vi "MultipleDbsPanelModel-GFV.vi"(8 "error in (no error)":errorcluster, 10 "Data in":variant, 11 "Enum":T1) -> (0 "error out":errorcluster, 3 "Data out":variant)   [LabVIEW 2013]
doc: "Use this template to build a VI to use as a subVI."
uses:
  TypeDef/MultipleFileDataModel.ctl
  TypeDef/MultipleFilesModelOutput.ctl
  TypeDef/MultipleFilesModelInput.ctl
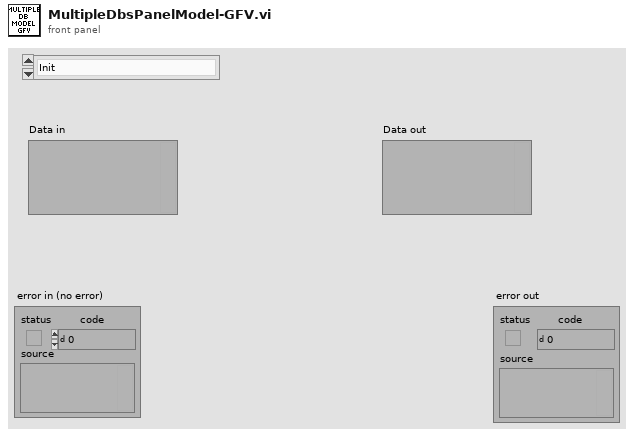
[diagram p1: front panel]
types:
  T1 = typedef "MultipleFileDataModel.ctl" = enum16{"Init", "Get Input Data", "Get Output Data", "Save Output Data", "Save Input Data"}
  T2 = typedef "MultipleFilesModelOutput.ctl" = cluster{"Ramp Pattern":dbl[], dbl[]}
  T3 = typedef "MultipleFilesModelInput.ctl" = cluster{"Min Diameter (µm)":dbl, "Max Diameter (µm)":dbl, "FilterDropletsFrozeBelow":dbl, "Temperature offset for Calibration":dbl, "BinSizeDeg":dbl}
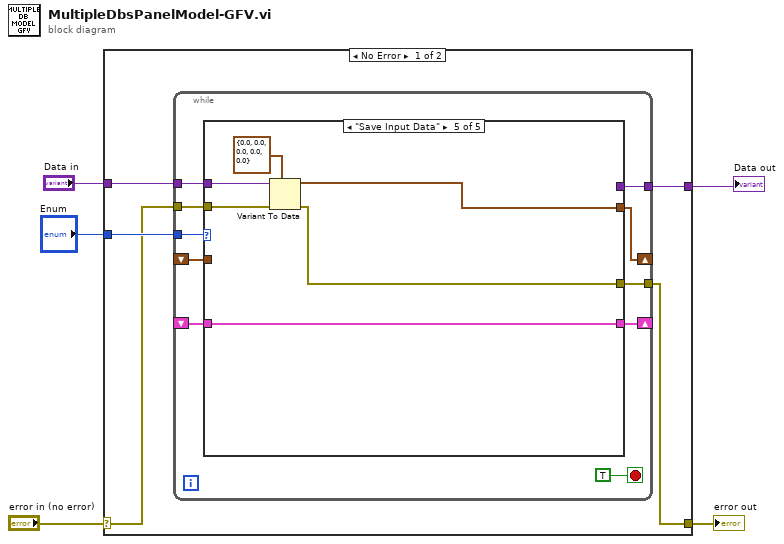
[diagram p0: block diagram]
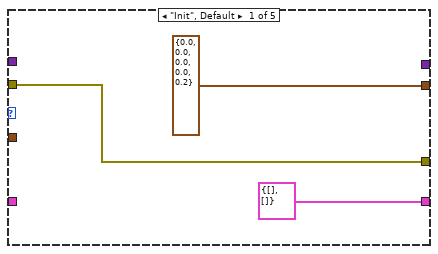
[diagram p2: hidden frame]
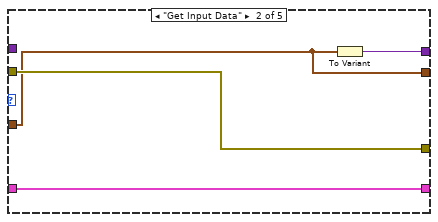
[diagram p3: hidden frame]
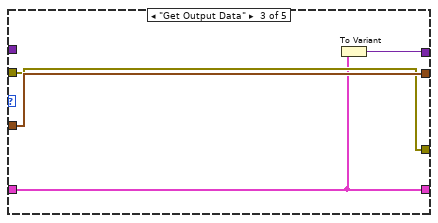
[diagram p4: hidden frame]
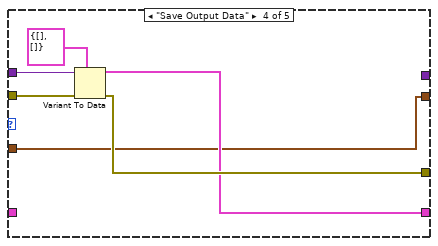
[diagram p5: hidden frame]
diagram:
  n1 = case shown="No Error" "error in (no error)" {
    selector: "error in (no error)" -> [w8 w44]
    tunnel: [w7 w44] -> w4
    tunnel: "Enum" -> [w10 _]
    tunnel: "Data in" -> [w9 _]
    tunnel: [w6 _] -> w1
    frame No Error {
      n2 = while {
        tunnel: w10 -> [w19]
        shift-right: [w18] -> _
        shift-left: _ -> [w14]
        tunnel: w9 -> [w17]
        tunnel: w8 -> [w16]
        tunnel: [w15] -> w7
        tunnel: [w13] -> w6
        shift-right: [w12] -> _
        shift-left: _ -> [w11]
        stop <- TRUE stop-if-true
        n3 = case shown="\"Save Input Data\"" w19 {
          tunnel: [T3 {"Min Diameter (µm)"=0.0, "Max Diameter (µm)"=0.0, "FilterDropletsFrozeBelow"=0.0, "Temperature offset for Calibration"=0.0, "BinSizeDeg"=0.2} w25 w31 w32 w39] -> w18
          tunnel: w17 -> [_ _ _ w37 w43]
          tunnel: w16 -> [w22 w26 w30 w36 w42]
          tunnel: [w22 w26 w30 w35 w41] -> w15
          tunnel: w14 -> [_ w25 w31 w32 _]
          tunnel: [_ w27 w29 _ _] -> w13
          tunnel: [T2 {"Ramp Pattern"=[], []} w24 w28 w33 w38] -> w12
          tunnel: w11 -> [_ w24 w28 _ w38]
          frame "Init", Default {
          }
          frame "Get Input Data" {
            n4 = To Variant(anything=w25) -> (Variant=w27:variant)
          }
          frame "Get Output Data" {
            n5 = To Variant(anything=w28) -> (Variant=w29:variant)
          }
          frame "Save Output Data" {
            n6 = Variant To Data(error in=w36, type=T2 {"Ramp Pattern"=[], []}, Variant=w37) -> (data=w33:T2, error out=w35:errorcluster)
          }
          frame "Save Input Data" {
            n7 = Variant To Data(error in=w42, type=T3 {"Min Diameter (µm)"=0.0, "Max Diameter (µm)"=0.0, "FilterDropletsFrozeBelow"=0.0, "Temperature offset for Calibration"=0.0, "BinSizeDeg"=0.0}, Variant=w43) -> (data=w39:T3, error out=w41:errorcluster)
          }
        }
      }
    }
    frame Error {
    }
  }
  "error out" <- w4
  "Data out" <- w1
